vi "Test Run VI Job.vi"() -> ()   [LabVIEW 2014]
uses:
  Core/Shared/Controls/Run VI - STYP.ctl
  Core/Shared/Classes/Status Updater/Status Updater.lvclass/Status Updater.ctl
  Core/LabVIEW CI Service/Classes/Job/Job.lvclass/Job.ctl
  Core/LabVIEW CI Service/Extensions/Run VI/Run VI/Run VI.lvclass
  Core/Shared/Classes/Status Updater/Status Updater.lvclass
  Core/LabVIEW CI Service/Classes/Job/Job.lvclass
panel:
  out "Results":T1 {"Status" items=["Service Error"=504, "Abort"=503, "Fail"=500, "Pass"=200]}
  out "Progress Percents":u32[](array[numeric])
  out "Steps":string[](array[string])
  in  "Executor Number":i32
  in  "VI Path":path=path "P:/alsmith/Sales/users/ACS/LabVIEW Continuous Integration/Jenkins Sample Project/Run VI Golden DUT.vi"
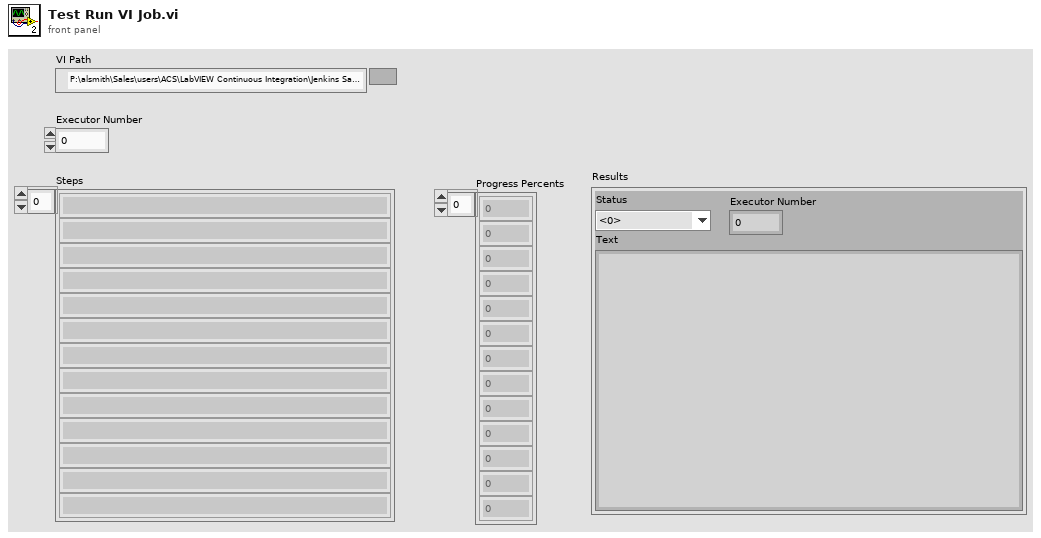
[diagram p1: front panel]
types:
  T1 = cluster{"Status":u16, "Text":string, "Executor Number":i32}
  T2 = typedef "Run VI - STYP.ctl" = cluster{"Executor_Number":string, "VI_Path":string, "Wait_Until_Done":bool}
  T3 = cluster{"Event Registration Refnum":refnum<event-registration>, "Event Registration Refnum":refnum<event-registration>}
  T4 = typedef "Job Results - STYP.ctl" = cluster{"Status":u16, "Text":string, "Executor Number":i32}
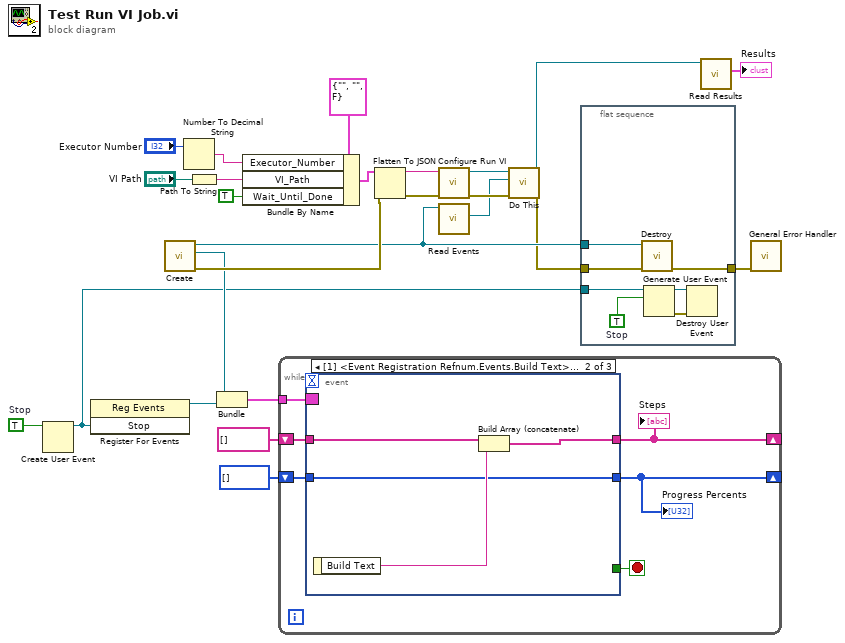
[diagram p0: block diagram]
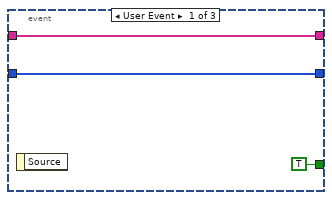
[diagram p2: hidden frame]
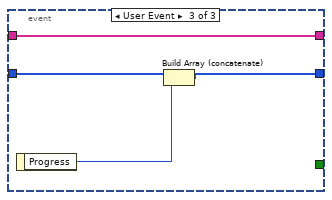
[diagram p3: hidden frame]
diagram:
  w19 = TRUE  # Stop
  n1 = Create User Event(user event datatype=w19) -> (user event=w15:refnum<user-event>)  [unwired: 1 in, 1 out]
  n2 = register-events(w15) -> (reference out=w16:refnum<event-registration>)  [unwired: 2 in, 1 out]
  n3 = call "Create.vi"() -> ("error out"=w20:errorcluster, "Event Registration Refnum"=w18:refnum<event-registration>, "Status Updater out"=w10:refnum<class "Status Updater.lvclass">)  [unwired: 9 in]
  n4 = Number To Decimal String(number="Executor Number") -> (decimal integer string=w24:string)  [unwired: 1 in]
  n5 = Path To String(path="VI Path") -> (string=w23:string)
  n6 = Bundle("Event Registration Refnum"=w18, "Event Registration Refnum"=w16) -> (w17:T3)  [unwired: 1 in]
  n7 = Bundle By Name(cluster=T2 {"Executor_Number"="", "VI_Path"="", "Wait_Until_Done"=FALSE} ("Run VI"), "Executor_Number"=w24, "VI_Path"=w23, "Wait_Until_Done"=TRUE) -> (w25:T2)
  n8 = while {
    tunnel: w17 -> [w31]
    shift-right: [w27] -> _
    shift-left: string[] [] -> [w29]
    shift-right: [w26] -> _
    shift-left: u32[] [] -> [w28]
    stop <- w30 stop-if-true
    n9 = event shown="[1] <Event Registration Refnum.Events.Build Text>: User Event" {
      selector: w31 -> [_ _ _]
      dyn-events: _ -> [_ _ _]
      timeout: _ -> [_ _ _]
      tunnel: [TRUE _ _] -> w30
      tunnel: w29 -> [w33 w38 w42]
      tunnel: [w33 w37 w42] -> w27
      tunnel: w28 -> [w32 w35 w41]
      tunnel: [w32 w35 w40] -> w26
      event User Event {
        n10 = event-data() -> ()  [unwired: 1 in, 1 out]
      }
      event User Event {
        n11 = event-data() -> ("Build Text"=w36:string)  [unwired: 1 in]
        n12 = Build Array (concatenate)(w38, w36) -> (w37:string[])
      }
      event User Event {
        n13 = event-data() -> ("Progress"=w39:u32)  [unwired: 1 in]
        n14 = Build Array (concatenate)(w41, w39) -> (w40:u32[])
      }
    }
    "Steps" <- w27
    "Progress Percents" <- w26
  }
  n15 = Flatten To JSON(anything=w25, error in (no error)=w20) -> (JSON string=w8:string, 11:w9:errorcluster)  [unwired: 1 in]
  n16 = call "Configure Run VI.vi"("error in (no error)"=w9, "JSON string"=w8) -> ("error out"=w6:errorcluster, "Run VI Out"=w4:refnum<class "Run VI.lvclass">)  [unwired: 8 in]
  n17 = call "Read Events.vi"("Status Updater in"=w10) -> ("Status Events"=w5:refnum<class "Status Events.lvclass">)  [unwired: 10 in]
  n18 = call-dynamic "Do This.vi"("error in (no error)"=w6, "Status Events"=w5, "Run VI in"=w4) -> ("error out"=w2:errorcluster, "Run VI out"=w3:refnum<class "Run VI.lvclass">)  [unwired: 7 in]
  n19 = flat-sequence {
    tunnel: w10 -> [w49]
    tunnel: w2 -> [w48]
    tunnel: w15 -> [w46]
    tunnel: [w45] -> w12
    frame #0 {
      w47 = TRUE  # Stop
      n20 = call "Destroy.vi"("error in (no error)"=w48, "Status Updater in"=w49) -> ("error out"=w45:errorcluster)  [unwired: 9 in]
      n21 = Generate User Event(user event=w46, event data cluster=w47) -> (user event out=w43:refnum<user-event>, error out=w44:errorcluster)  [unwired: 2 in]
      n22 = Destroy User Event(user event=w43, error in=w44) -> ()  [unwired: 1 out]
    }
  }
  n23 = call "Read Results.vi"("Job in"=w3) -> ("Results"=→"Results":T4)  [unwired: 10 in]
  n24 = call <vilib>:"General Error Handler.vi"("error in (no error)"=w12) -> ()  [unwired: 10 in, 5 out]
